vi "AR Order Estimation.vi"() -> ()   [LabVIEW 2023]
doc: "This example shows how to obtain AR model order of a univariate time series using the TSA AR Modeling Order VI.\n\n<b>Instructions:</b>\n1) Run this VI.\n2) Set the coefficients for the IIR filter.\n3) Select the method and range to search the AR order for the simulated time series.\n4) Observe the criterion function and the estimated optimal order."
uses:
  <vilib>/Analysis/3filter.llb/IIR Filter (DBL).vi
  <vilib>/addons/Time Series Analysis/Modeling and Prediction.llb/TSA AR Modeling Order (Array).vi
  <vilib>/addons/_Advanced Signal Processing/NI_AdvSigProcTSA.lvlib
  <vilib>/Analysis/NI_AALBase.lvlib
panel:
  out "Time Series from the Simulated System":dbl[](graph)
  in  "Reverse coefficients":dbl[](array[numeric])=[1.0, 1.5, 0.7, 0.1]
  in  "stop":bool
  in  "Order range":cluster{"Low":i32, "High":i32}={"Low"=1, "High"=10}
  in  "Method":i32(ring)=3 items=["Final Prediction Error"=0, "Akaike Information"=1, "Bayesian Information"=2, "Minimal Description Length"=3, "Phi Criterion"=4, "-"=-1, "Partial Correlation Function"=6]
  out "Criterion Function":T1(graph)
  out "Estimated optimal AR order":i32=3
  # "Overview: Shows how to obtain AR model order of a univariate time series using the TSA AR Modeling Order VI.\nRequirements: LabVIEW Full Development System, Advanced Signal Processing Toolkit\nInstructions: \n1. Run this VI.\n2. Set the coefficients for the IIR filter.\n3. Select the method and range to search the AR order for the simulated time series.\n4. Observe the criterion function and the estimated optimal order.   \n5. Click Stop to stop the VI."
  # "Simulated System (IIR Filter)"
  # "AR Order Estimation Settings"
  # "The first element of Reverse coefficients must be 1."
  # "Forward coefficients = [1]"
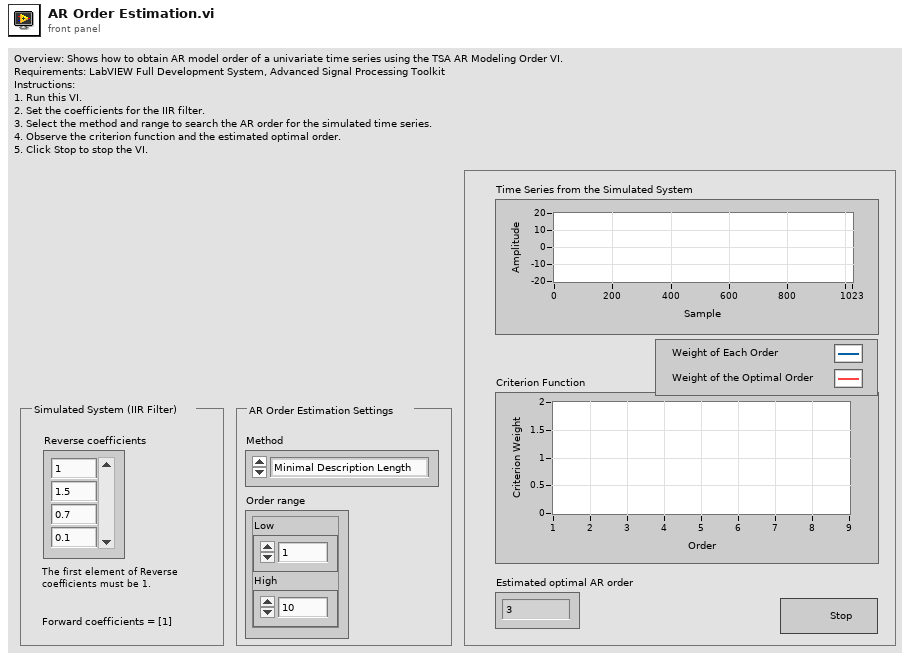
[diagram p1: front panel]
types:
  T1 = cluster{"order":i32[], "prediction error":dbl[]}[]
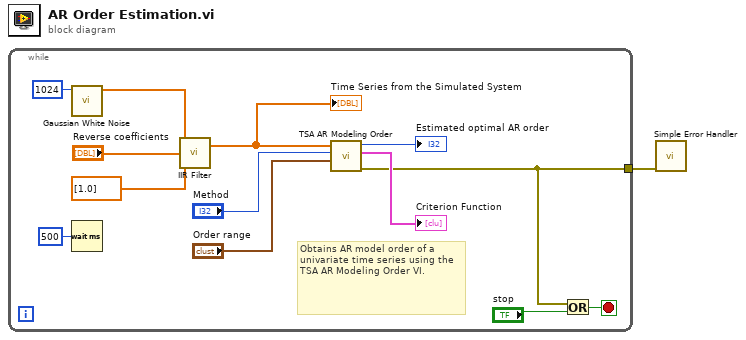
[diagram p0: block diagram]
diagram:
  n1 = while {
    tunnel: [w2] -> w1
    stop <- w4 stop-if-true
    # "Obtains AR model order of a univariate time series using the TSA AR Modeling Order VI."
    n2 = call <vilib>:"Gaussian White Noise.vi"("samples"=1024) -> ("Gaussian noise pattern"=w14:dbl[])  [unwired: 9 in, 1 out]
    n3 = Wait (ms)(milliseconds to wait=u32 500 ("millisecond multiple")) -> ()  [unwired: 1 out]
    n4 = call-poly <vilib>:"IIR Filter.vi"("Forward Coefficients"=dbl[] [1.0], "Reverse Coefficients"="Reverse coefficients", "X"=w14) -> ("Filtered X"=w6:dbl[])  [unwired: 1 in, 1 out]
    "Time Series from the Simulated System" <- w6
    n5 = call-poly <vilib>:"TSA AR Modeling Order.vi"("order range"="Order range", "method"="Method", "Xt"=w6) -> ("error out"=w2:errorcluster, "criterion function"=→"Criterion Function":T1, "optimal AR order"=→"Estimated optimal AR order":i32)  [unwired: 2 in, 4 out]
    n6 = Or(x=w2, y="stop") -> (x .or. y?=w4:bool)
  }
  n7 = call <vilib>:"Simple Error Handler.vi"("error in (no error)"=w1) -> ()  [unwired: 1 in, 8 out]
